vi "Update Dependency.vi"(6 "Level":string, 8 "error in (no error)":errorcluster, 9 "owned":bool, 10 "SMO":refnum<class "SMO.lvclass">, 11 "Attribute.Dependencies in":refnum<class "Attribute.Dependencies.lvclass">) -> (0 "error out":errorcluster, 3 "Attribute.Dependencies out":refnum<class "Attribute.Dependencies.lvclass">)   [LabVIEW 2013, in "Attribute.Dependencies.lvclass"]
uses:
  Attribute.Dependencies.lvclass
  SMO/SMO.lvclass
  DependencyAttr--Cluster.ctl
  Attribute.Dependencies.lvclass/Attribute.Dependencies.ctl
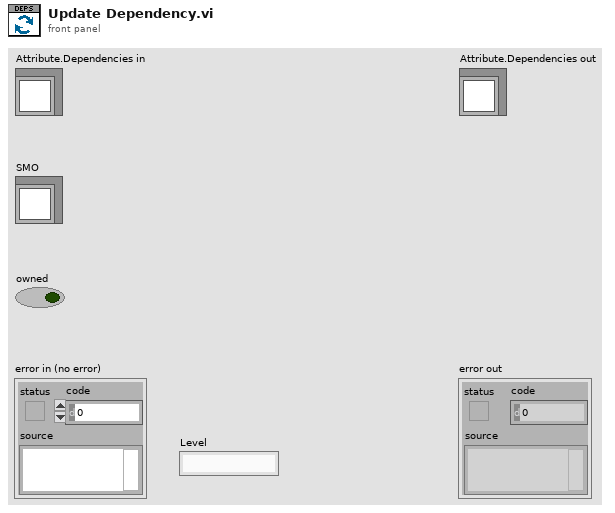
[diagram p1: front panel]
types:
  T1 = typedef "Attribute.Dependencies.lvclass/DependencyAttr--Cluster.ctl" = cluster{"Name":string, "GUID":string, "owned":bool, "shared":bool, "Level":string, "SMO":refnum<class "SMO.lvclass">}
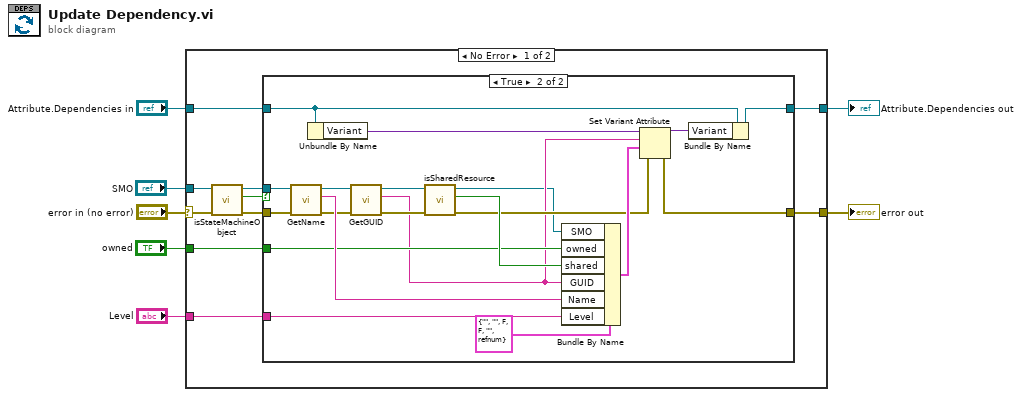
[diagram p0: block diagram]
diagram:
  n1 = case shown="No Error" "error in (no error)" {
    selector: "error in (no error)" -> [w11 w41]
    tunnel: [w10 w41] -> w6
    tunnel: [w17 w40] -> w4
    tunnel: "Attribute.Dependencies in" -> [w16 w40]
    tunnel: "SMO" -> [w15 _]
    tunnel: "owned" -> [w9 _]
    tunnel: "Level" -> [w8 _]
    frame No Error {
      n2 = call "isStateMachineObject.vi"("error in (no error)"=w11, "SMO"=w15) -> ("error out"=w12:errorcluster, "is SMO?"=w13:bool, "SMO out"=w14:refnum<class "SMO.lvclass">)  [unwired: 7 in]
      n3 = case shown="True" w13 {
        tunnel: [w19 w34] -> w17
        tunnel: w16 -> [w19 w33]
        tunnel: w14 -> [_ w27]
        tunnel: w12 -> [w18 w26]
        tunnel: [w18 w24] -> w10
        tunnel: w9 -> [_ w23]
        tunnel: w8 -> [_ w21]
        frame False {
        }
        frame True {
          n4 = call "GetName.vi"("error in (no error)"=w26, "SMO"=w27) -> ("error out"=w29:errorcluster, "Name"=w35:string, "SMO out"=w39:refnum<class "SMO.lvclass">)  [unwired: 7 in]
          n5 = Unbundle By Name(w33) -> ("Variant"=w31:variant)
          n6 = call "GetGUID.vi"("error in (no error)"=w29, "SMO"=w39) -> ("error out"=w28:errorcluster, "GUID"=w22:string, "SMO out"=w38:refnum<class "SMO.lvclass">)  [unwired: 7 in]
          n7 = call "isSharedResource.vi"("error in (no error)"=w28, "SMO in"=w38) -> ("error out"=w25:errorcluster, "shared resource"=w36:bool, "SMO out"=w20:refnum<class "SMO.lvclass">)  [unwired: 7 in]
          n8 = Bundle By Name(cluster=T1 {"Name"="", "GUID"="", "owned"=FALSE, "shared"=FALSE, "Level"="", "SMO"=refnum} ("Dependency"), "SMO"=w20, "owned"=w23, "shared"=w36, "GUID"=w22, "Name"=w35, "Level"=w21) -> (w30:T1)
          n9 = Set Variant Attribute(Variant=w31, name=w22, value=w30, error in=w25) -> (Variant out=w32:variant, error out=w24:errorcluster)  [unwired: 1 out]
          n10 = Bundle By Name(cluster=w33, "Variant"=w32) -> (w34:refnum<class "Attribute.Dependencies.lvclass">)
        }
      }
    }
    frame Error {
    }
  }
  "error out" <- w6
  "Attribute.Dependencies out" <- w4
